vi "Update Operating Mode.vi"(10 "UTP IO Session in":T1, 11 "Sequence Context In":refnum<k7>) -> ()   [LabVIEW 2023]
uses:
  <vilib>/Noffz/UTP IO/UTP IO Library/Typedefs/Session Handle.ctl
  <vilib>/Noffz/UTP IO/UTP IO Library/UTP IO Pool Session.lvclass
  <vilib>/Noffz/UTP IO/UTP IO Library/methods/poly/plc/Read PLC Variable (I16).vi
  <vilib>/addons/TestStand/_TSUtility.llb/TestStand - Set Property Value (Number {Signed 16-bit Integer}).vi
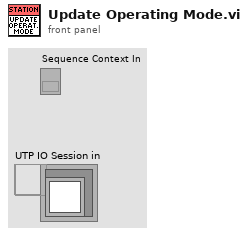
[diagram p1: front panel]
types:
  T1 = typedef "UTP IO Library.lvlib/UTP IO Pool Session.lvclass/Session Handle.ctl" = refnum<data-value>
  T2 = typedef "TestStand - Status Monitor.ctl" = cluster{"Sequence Context":refnum<k7>, "Execution":refnum<k7>, "Termination Monitor":refnum<k7>}
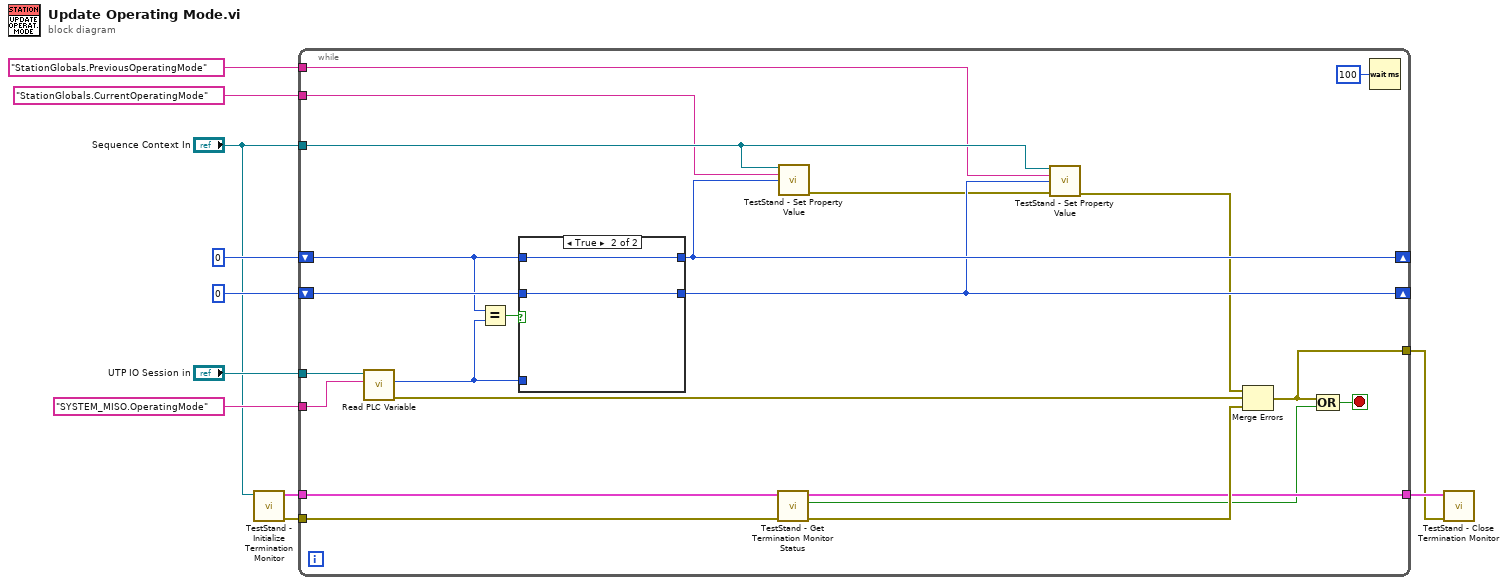
[diagram p0: block diagram]
diagram:
  n1 = call <vilib>:"TestStand - Initialize Termination Monitor.vi"("Sequence Context In"="Sequence Context In") -> ("error out"=w6:errorcluster, "Status Monitor Out"=w5:T2)  [unwired: 9 in]
  n2 = while {
    tunnel: "UTP IO Session in" -> [w33]
    tunnel: "SYSTEM_MISO.OperatingMode" ("variable name") -> [w32]
    shift-right: [w25] -> _
    shift-left: i16 0 ("value") -> [w27]
    shift-right: [w24] -> _
    shift-left: i16 0 ("value") -> [w28]
    tunnel: "Sequence Context In" -> [w31]
    tunnel: w6 -> [w22]
    tunnel: w5 -> [w21]
    tunnel: [w17] -> w4
    tunnel: [w15] -> w3
    tunnel: "StationGlobals.CurrentOperatingMode" ("Lookup String") -> [w13]
    tunnel: "StationGlobals.PreviousOperatingMode" ("Lookup String") -> [w12]
    stop <- w16 stop-if-true
    n3 = call-poly <vilib>:"Read PLC Variable.vi"("variable name"=w32, "UTP IO Session in"=w33) -> ("error out"=w19:errorcluster, "value"=w29:i16)  [unwired: 7 in, 1 out]
    n4 = Equal?(x=w27, y=w29) -> (x = y?=w30:bool)
    n5 = case shown="True" w30 {
      tunnel: w29 -> [w34 _]
      tunnel: [w34 w36] -> w25
      tunnel: [w35 w37] -> w24
      tunnel: w28 -> [_ w37]
      tunnel: w27 -> [w35 w36]
      frame False {
      }
      frame True {
      }
    }
    n6 = call <vilib>:"TestStand - Get Termination Monitor Status.vi"("error in (no error)"=w22, "Status Monitor In"=w21) -> ("error out"=w18:errorcluster, "Terminating or Aborting"=w14:bool, "Status Monitor Out"=w17:T2)  [unwired: 7 in]
    n7 = call-poly <vilib>:"TestStand - Set Property Value.vi"("Sequence Context In"=w31, "Lookup String"=w13, "New Value"=w25) -> ("error out"=w23:errorcluster)  [unwired: 11 in, 1 out]
    n8 = call-poly <vilib>:"TestStand - Set Property Value.vi"("Sequence Context In"=w31, "Lookup String"=w12, "New Value"=w24, "error in (no error)"=w23) -> ("error out"=w20:errorcluster)  [unwired: 10 in, 1 out]
    n9 = Merge Errors(w20, w19, w18) -> (w15:errorcluster)
    n10 = Compound Arithmetic op=OR(w15, w14) -> (w16:bool)
    n11 = Wait (ms)(milliseconds to wait=u32 100) -> ()  [unwired: 1 out]
  }
  n12 = call <vilib>:"TestStand - Close Termination Monitor.vi"("error in (no error)"=w3, "Status Monitor In"=w4) -> ()  [unwired: 9 in, 1 out]
